vi "ParseNewTracepoint.vi"(8 "error in (no error)":errorcluster, 11 "message body":variant) -> (0 "error out":errorcluster, 3 "tracepoint":string)   [LabVIEW 2014, in "TraceLogger.lvlib"]
uses:
  <vilib>/addons/TraceLogger/TraceLogger.lvlib
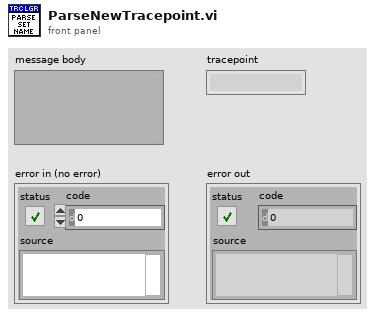
[diagram p1: front panel]
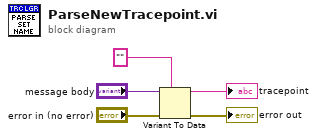
[diagram p0: block diagram]
diagram:
  n1 = Variant To Data(error in="error in (no error)", type="" ("instance name"), Variant="message body") -> (data=→"tracepoint":string, error out=→"error out":errorcluster)
